vi "Write Report File.vi"(8 "error in (no error)":errorcluster, 10 "Test Report":refnum<class "Test Report.lvclass">, 11 "Test Assert Factory in":refnum<class "Test Assert Factory.lvclass">) -> (0 "error out":errorcluster, 3 "Test Assert Factory out":refnum<class "Test Assert Factory.lvclass">)   [LabVIEW 2009, in "Caraya.lvlib" / "Test Assert Factory.lvclass"]
uses:
  Test Assert Factory.lvclass
  Test Report/Test Report.lvclass
  Test Assert Factory.lvclass/Test Assert Factory.ctl
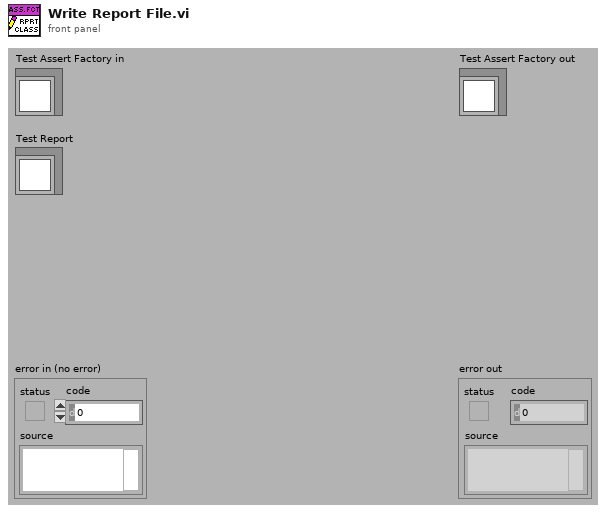
[diagram p1: front panel]
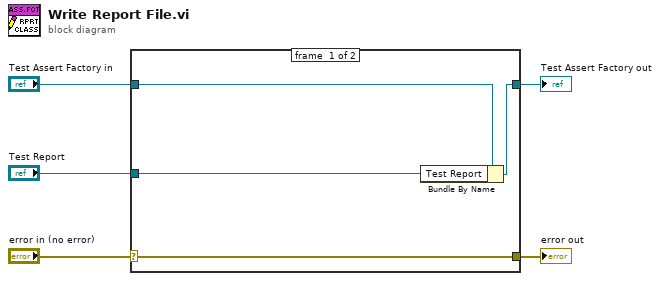
[diagram p0: block diagram]
diagram:
  n1 = case shown="No Error" "error in (no error)" {
    selector: "error in (no error)" -> [w9 w10]
    tunnel: [w9 w10] -> w4
    tunnel: [w7 w11] -> w2
    tunnel: "Test Assert Factory in" -> [w8 w11]
    tunnel: "Test Report" -> [w6 _]
    frame #0 {
      n2 = Bundle By Name(cluster=w8, "Test Report"=w6) -> (w7:refnum<class "Test Assert Factory.lvclass">)
    }
    frame #1 {
    }
  }
  "error out" <- w4
  "Test Assert Factory out" <- w2
